vi "startNextCycle.vi"(8 "error in (no error)":errorcluster, 11 "Model in":refnum<class "Model.lvclass">) -> (0 "error out":errorcluster, 3 "Model out":refnum<class "Model.lvclass">)   [LabVIEW 2015]
uses:
  ApplicationElements/TestMonitor/TestMonitor.lvclass
  UserEvents/UserEvents.lvclass
  ApplicationElements/Log/TestDataLog/TestDataLog.lvclass
  Model.lvclass
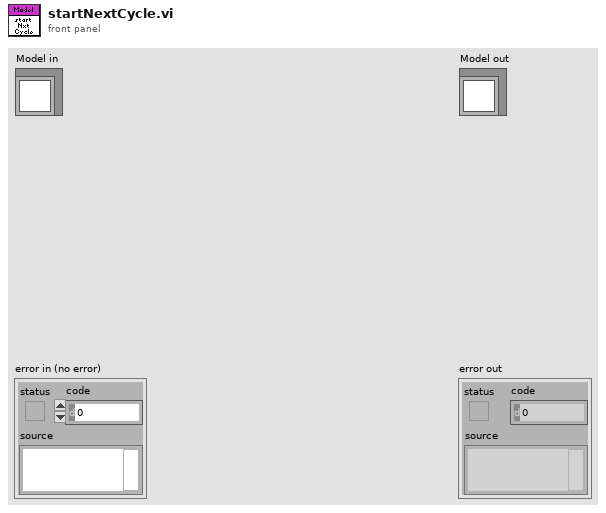
[diagram p1: front panel]
types:
  T1 = typedef "M1M3SSSTypedefs.lvlib/TestStatus.ctl" = cluster{"activeCycle":u32, "activeProfileStep":u32, "demandedCycles":u32, "demandedProfileSteps":u32}
  T2 = typedef "M1M3SSSTypedefs.lvlib/PubDataEvents.ctl" = cluster{"State":refnum<user-event>, "ErrorCode":refnum<user-event>, "OutputData":refnum<user-event>, "InputData":refnum<user-event>, "ControllerData":refnum<user-event>, "TestStatus":refnum<user-event>, "LogPath":refnum<user-event>, "StiffnessData":refnum<user-event>, "PreconditioningCycle":refnum<user-event>}
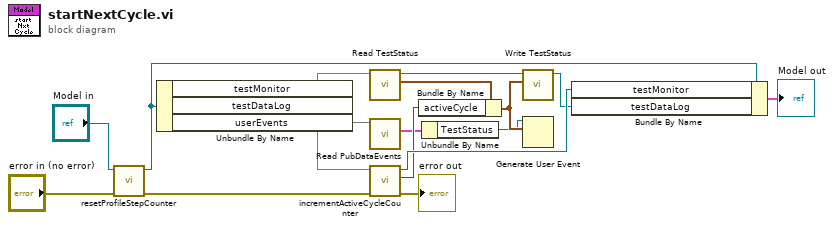
[diagram p0: block diagram]
diagram:
  n1 = call "resetProfileStepCounter.vi"("error in (no error)"="error in (no error)", "Model in"="Model in") -> ("error out"=w16:errorcluster, "Model out"=w14:refnum<class "Model.lvclass">)  [unwired: 8 in]
  n2 = Unbundle By Name(w14) -> ("testMonitor"=w17, "testDataLog"=w6, "userEvents"=w1)
  n3 = call "Read TestStatus.vi"("Logger in"=w6) -> ("TestStatus"=w9:T1, "Logger out"=w8:refnum<class "TestDataLog.lvclass">)  [unwired: 9 in]
  n4 = call "Read PubDataEvents.vi"("UserEvents in"=w1) -> ("PubDataEvents"=w3:T2)  [unwired: 9 in, 1 out]
  n5 = call "incrementActiveCycleCounter.vi"("error in (no error)"=w16, "TestMonitor in"=w17) -> ("error out"=→"error out":errorcluster, "activeCycle"=w7:u32, "TestMonitor out"=w10:refnum<class "TestMonitor.lvclass">)  [unwired: 7 in]
  n6 = Bundle By Name(cluster=w9, "activeCycle"=w7) -> (w4:T1)
  n7 = Unbundle By Name(w3) -> ("TestStatus"=w2:refnum<user-event>)
  n8 = call "Write TestStatus.vi"("TestStatus"=w4, "Logger in"=w8) -> ("Logger out"=w5:refnum<class "TestDataLog.lvclass">)  [unwired: 9 in]
  n9 = Generate User Event(user event=w2, event data cluster=w4) -> ()  [unwired: 2 in, 2 out]
  n10 = Bundle By Name(cluster=w14, "testMonitor"=w10, "testDataLog"=w5) -> (→"Model out":cluster{})
